vi "accept tls server.vi"(8 "error in":errorcluster, 11 "client":u64) -> (0 "error out":errorcluster, 2 "lvsocket":u64, 3 "connection":u64)   [LabVIEW 2016, in "lv tls dll.lvlib"]
uses:
  lv tls dll.lvlib
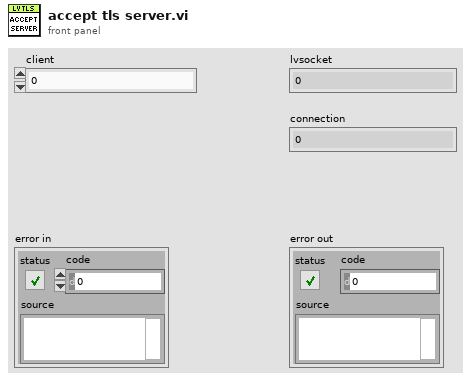
[diagram p1: front panel]
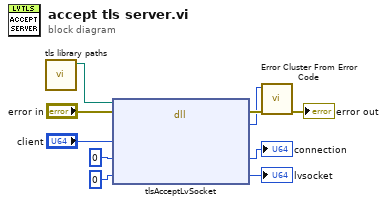
[diagram p0: block diagram]
diagram:
  n1 = call "tls library paths.vi"() -> ("lvtls"=w8:path)  [unwired: 8 in, 3 out]
  n2 = dll-call lib="C:/Users/IEUser/Desktop/tlssimple/lvlibtls.dll" fn="tlsAcceptLvSocket"(path in=w8, error in="error in", "server"="client", "connection"=u64 0 ("lvsocket"), "lvsocket"=u64 0) -> (error out=w10:errorcluster, "err"=w9:i32, "connection"=→"connection":u64, "lvsocket"=→"lvsocket":u64)  [unwired: 2 in, 1 out]
  n3 = call <vilib>:"Error Cluster From Error Code.vi"("error in (no error)"=w10, "error code (0)"=w9) -> ("error out"=→"error out":errorcluster)  [unwired: 7 in]
